vi "leitura_configuracao_valvulas_adq.vi"() -> (2 "Valvulas":T1)   [LabVIEW 2019]
uses:
  <vilib>/Utility/file.llb/Read Delimited Spreadsheet (DBL).vi
panel:
  in  "Valvulas 2":T1
  out "first row":dbl[](array[numeric])
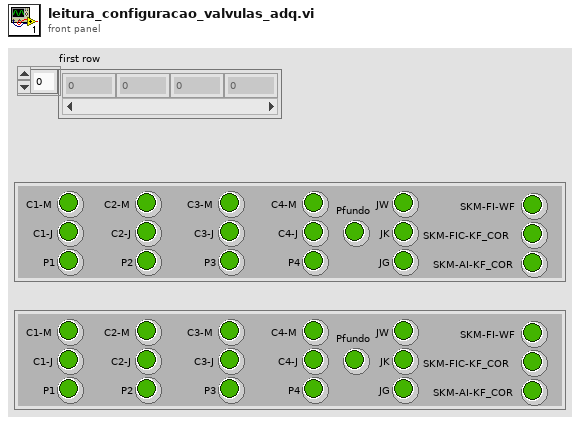
[diagram p1: front panel]
types:
  T1 = cluster{"C1-M":bool, "C1-J":bool, "P1":bool, "C2-M":bool, "C2-J":bool, "P2":bool, "C3-M":bool, "C3-J":bool, "P3":bool, "C4-M":bool, "C4-J":bool, "P4":bool, "Pfundo":bool, "JW":bool, "JK":bool, "JG":bool, "SKM-FI-WF":bool, "SKM-FIC-KF_COR":bool, "SKM-AI-KF_COR":bool}
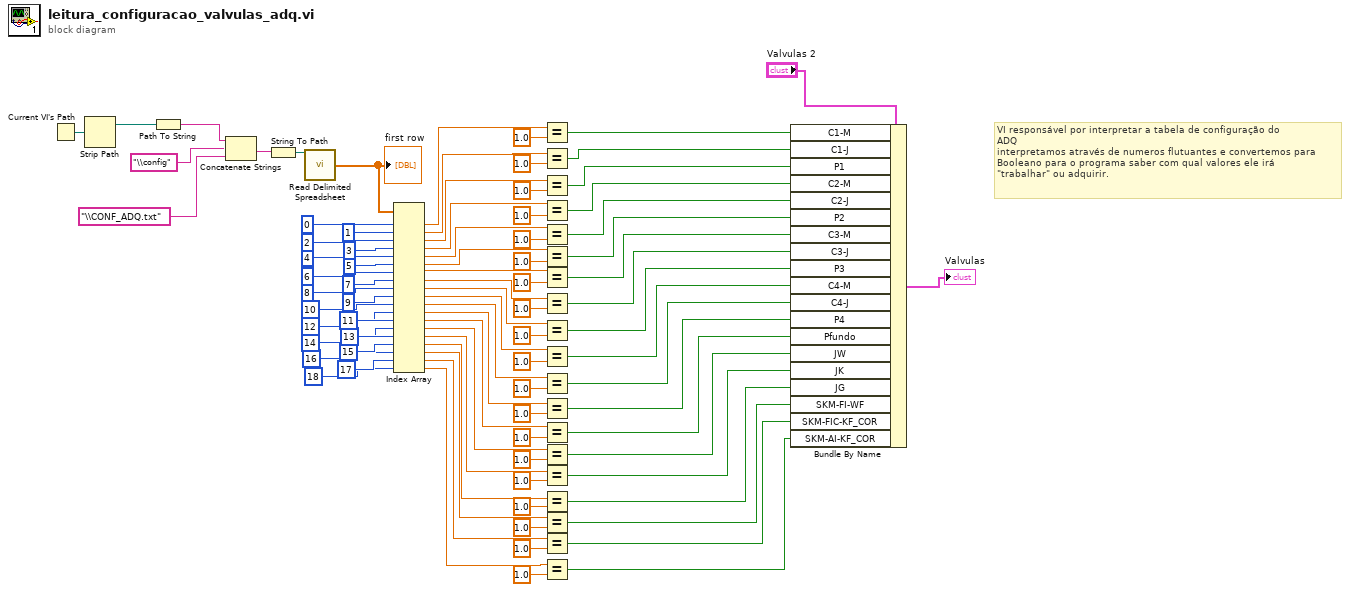
[diagram p0: block diagram]
diagram:
  # "VI responsável por interpretar a tabela de configuração do \nADQ\ninterpretamos através de numeros flutuantes e convertemos para\nBooleano para o programa saber com qual valores ele irá\n\"trabalhar\" ou adquirir."
  n1 = Current VI's Path() -> (path=w85:path)
  n2 = Strip Path(path=w85) -> (stripped path=w2:path)  [unwired: 1 out]
  n3 = Path To String(path=w2) -> (string=w86:string)
  n4 = Concatenate Strings(w86, "\\config" ("string"), "\\CONF_ADQ.txt" ("string")) -> (w84:string)
  n5 = String To Path(string=w84) -> (path=w82:path)
  n6 = call-poly <vilib>:"Read Delimited Spreadsheet.vi"("file path (dialog if empty)"=w82) -> ("first row"=w81:dbl[])  [unwired: 9 in, 5 out]
  "first row" <- w81
  n7 = Index Array(array=w81, index #1=0 ("index"), index #2=1 ("index"), index #3=2 ("index"), index #4=3 ("index"), index #5=4 ("index"), index #6=5 ("index"), index #7=6 ("index"), index #8=7 ("index"), index #9=8 ("index"), index #10=9 ("index"), index #11=10 ("index"), index #12=11 ("index"), index #13=12 ("index"), index #14=13 ("index"), index #15=14 ("index"), index #16=15 ("index"), index #17=16 ("index"), index #18=17 ("index"), index #19=18 ("index")) -> (element #1=w64:dbl, element #2=w47:dbl, element #3=w46:dbl, element #4=w45:dbl, element #5=w44:dbl, element #6=w43:dbl, element #7=w42:dbl, element #8=w41:dbl, element #9=w40:dbl, element #10=w39:dbl, element #11=w38:dbl, element #12=w37:dbl, element #13=w36:dbl, element #14=w35:dbl, element #15=w34:dbl, element #16=w33:dbl, element #17=w8:dbl, element #18=w7:dbl, element #19=w6:dbl)
  n8 = Equal?(x=w64, y=1.0) -> (x = y?=w62:bool)
  n9 = Equal?(x=w47, y=1.0) -> (x = y?=w32:bool)
  n10 = Equal?(x=w46, y=1.0) -> (x = y?=w31:bool)
  n11 = Equal?(x=w45, y=1.0) -> (x = y?=w30:bool)
  n12 = Equal?(x=w44, y=1.0) -> (x = y?=w29:bool)
  n13 = Equal?(x=w43, y=1.0) -> (x = y?=w28:bool)
  n14 = Equal?(x=w42, y=1.0) -> (x = y?=w27:bool)
  n15 = Equal?(x=w41, y=1.0) -> (x = y?=w26:bool)
  n16 = Equal?(x=w40, y=1.0) -> (x = y?=w25:bool)
  n17 = Equal?(x=w39, y=1.0) -> (x = y?=w24:bool)
  n18 = Equal?(x=w38, y=1.0) -> (x = y?=w23:bool)
  n19 = Equal?(x=w37, y=1.0) -> (x = y?=w22:bool)
  n20 = Equal?(x=w36, y=1.0) -> (x = y?=w21:bool)
  n21 = Equal?(x=w35, y=1.0) -> (x = y?=w19:bool)
  n22 = Equal?(x=w34, y=1.0) -> (x = y?=w18:bool)
  n23 = Equal?(x=w33, y=1.0) -> (x = y?=w17:bool)
  n24 = Equal?(x=w8, y=1.0) -> (x = y?=w5:bool)
  n25 = Equal?(x=w7, y=1.0) -> (x = y?=w4:bool)
  n26 = Equal?(x=w6, y=1.0) -> (x = y?=w3:bool)
  n27 = Bundle By Name(cluster="Valvulas 2", "C1-M"=w62, "C1-J"=w32, "P1"=w31, "C2-M"=w30, "C2-J"=w29, "P2"=w28, "C3-M"=w27, "C3-J"=w26, "P3"=w25, "C4-M"=w24, "C4-J"=w23, "P4"=w22, "Pfundo"=w21, "JW"=w19, "JK"=w18, "JG"=w17, "SKM-FI-WF"=w5, "SKM-FIC-KF_COR"=w4, "SKM-AI-KF_COR"=w3) -> (→"Valvulas":T1)
